vi "LWXPS_GatheringConfigurationGet.vi"(0 "XPS Reference IN":refnum<k24>, 11 "LabVIEW error IN":errorcluster) -> (4 "XPS Reference OUT":refnum<k24>, 6 "Returned error code":i32, 8 "Type":string[](array[string]), 10 "XPS Error String":string, 15 "LabVIEW error OUT":errorcluster)   [LabVIEW 2014]
uses:
  D:/XPSQ8_LabView_Library/Development/Source/Dll/Newport.XPS.CommandInterface.dll
  Dll/Newport.XPS.CommandInterface.dll
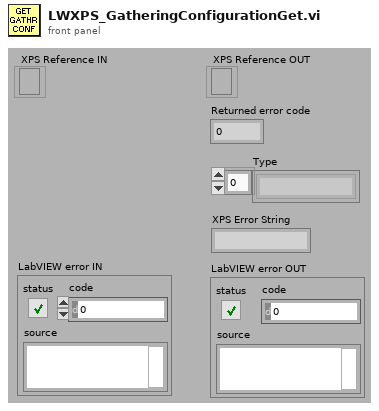
[diagram p1: front panel]
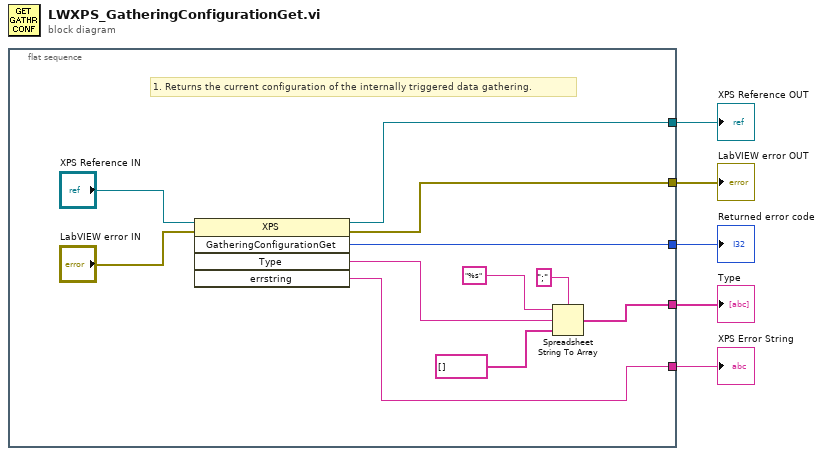
[diagram p0: block diagram]
diagram:
  n1 = flat-sequence {
    tunnel: [w11] -> w5
    tunnel: [w15] -> w4
    tunnel: [w14] -> w3
    tunnel: [w13] -> w2
    tunnel: [w6] -> w1
    frame #0 {
      # "1. Returns the current configuration of the internally triggered data gathering."
      n2 = invoke class="XPS" method="GatheringConfigurationGet"(reference="XPS Reference IN", error in="LabVIEW error IN") -> (reference out=w15:refnum<k24>, error out=w14:errorcluster, "GatheringConfigurationGet"=w13:i32, "Type"=w7:string, "errstring"=w11:string)  [unwired: 3 in]
      n3 = Spreadsheet String To Array(delimiter (Tab)=";" ("Delimiter (Tab)"), format string="%s" ("Format string"), spreadsheet string=w7, array type (2D Dbl)=string[] [] ("Type")) -> (array=w6:string[])
    }
  }
  "XPS Error String" <- w5
  "XPS Reference OUT" <- w4
  "LabVIEW error OUT" <- w3
  "Returned error code" <- w2
  "Type" <- w1
